vi "VisaReadExample2.vi"() -> ()   [LabVIEW 2016]
uses:
  <vilib>/Instr/_visa.llb/VISA Configure Serial Port (Instr).vi
panel:
  out "deleted portion":dbl[][](array[numeric])
  out "array w/ subset deleted":dbl[][](array[numeric])
  out "size(s)":i32
  out "PULSE":string="126526"
  in  "Upper Cut-Off":dbl=100.0
  in  "Lower Cut-Off":dbl=10.0
  in  "OK Button":bool
  out "Waveform Graph":dynamicdata(graph)
  in  "Array 2":dbl[](array[numeric])=array[6515 elements]
  in  "Array":dbl[](array[numeric])=array[6516 elements]
  out "substring 2":string="I"
  out "substring":string="126526"
  out "read buffer":string="I126526"
  in  "VISA resource name":refnum<visa-resource-name>="COM3"
  in  "stop":bool
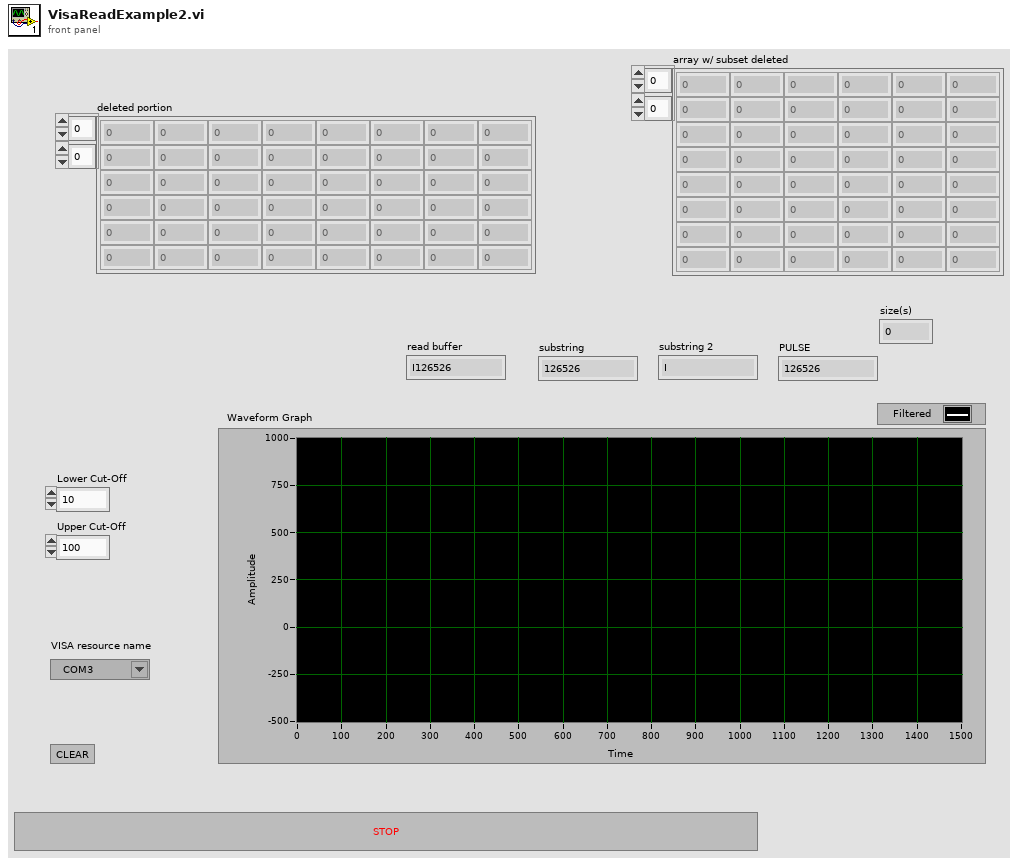
[diagram p1: front panel]
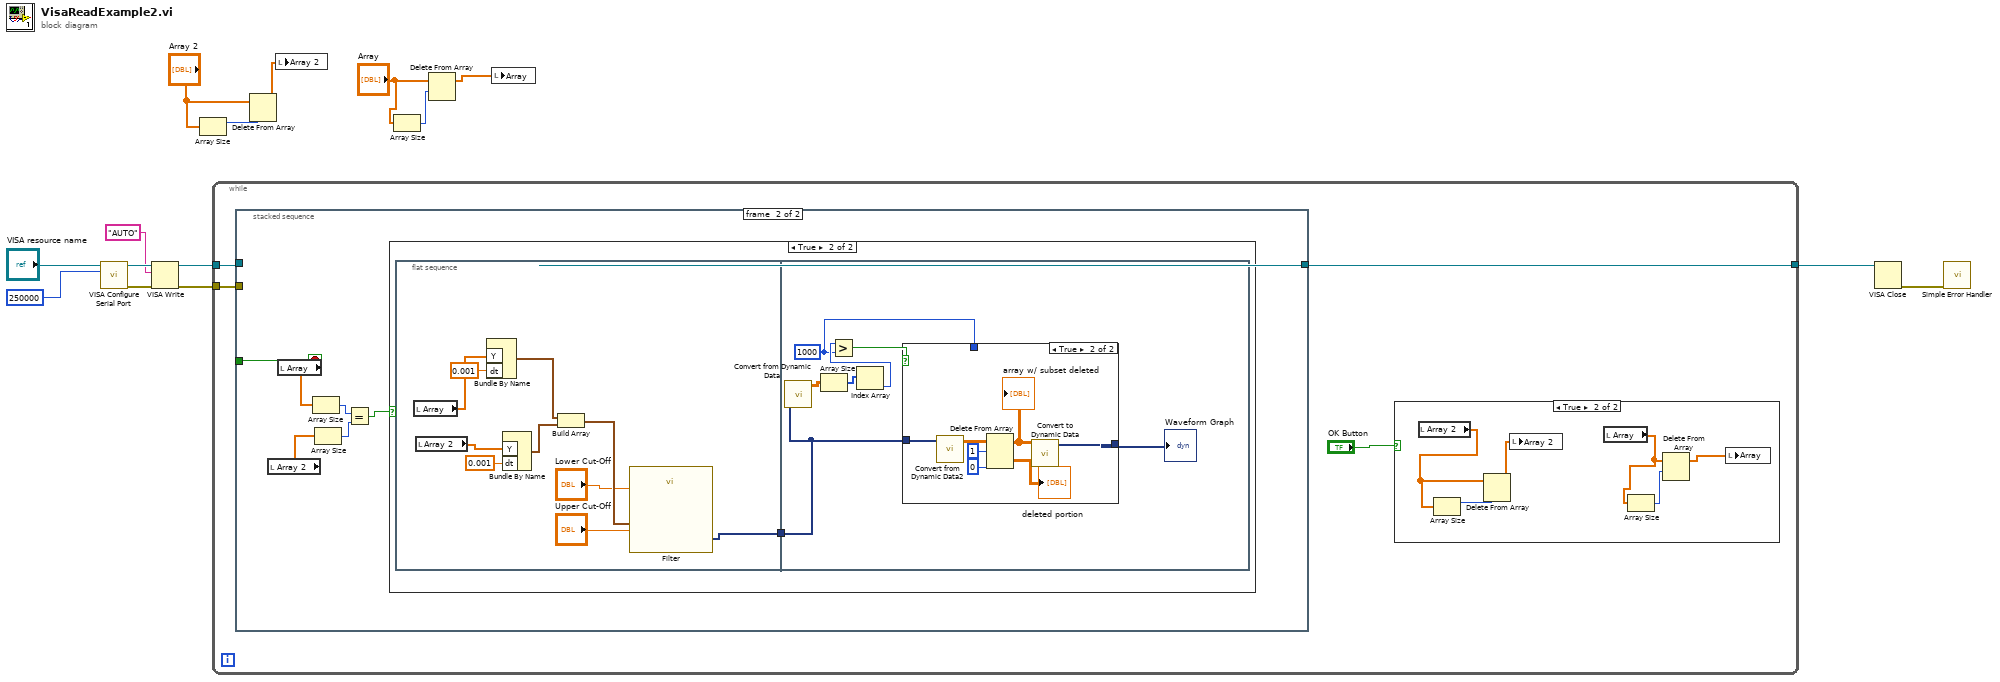
[diagram p0: block diagram]
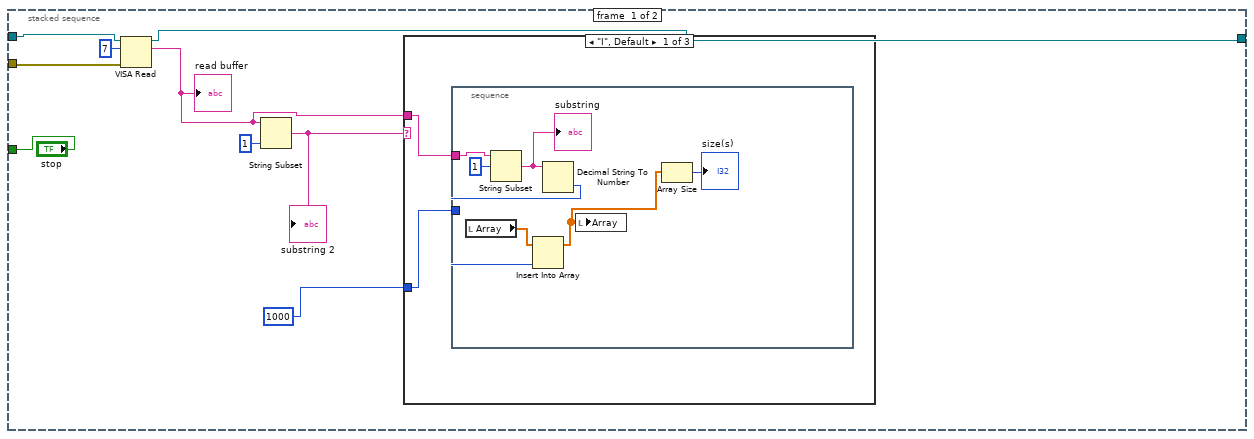
[diagram p3: hidden frame]
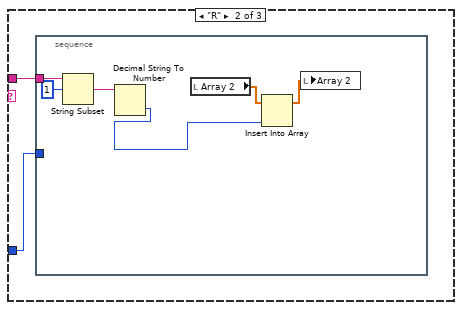
[diagram p4: hidden frame]
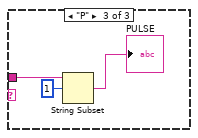
[diagram p5: hidden frame]
diagram:
  n1 = call-poly "VISA Configure Serial Port"("VISA resource name"="VISA resource name", "baud rate (9600)"=u32 250000) -> ("VISA resource name out"=w11:refnum<visa-resource-name>, "error out"=w9:errorcluster)  [unwired: 12 in]
  n2 = VISA Write(VISA resource name=w11, write buffer="AUTO", error in (no error)=w9) -> (VISA resource name out=w10:refnum<visa-resource-name>, error out=w8:errorcluster)  [unwired: 1 out]
  n3 = Array Size(array="Array 2") -> (size(s)=w3:i32)
  n4 = while {
    tunnel: [w19] -> w14
    tunnel: w10 -> [w18]
    tunnel: w8 -> [w17]
    stop <- w20 stop-if-true
    n5 = stacked-sequence {
      tunnel: ["stop" _] -> w20
      tunnel: [w34 _] -> w19
      tunnel: w18 -> [w32 _]
      tunnel: w17 -> [w29 _]
      frame #0 {
        n6 = VISA Read(VISA resource name=w32, byte count=u32 7, error in (no error)=w29) -> (VISA resource name out=w34:refnum<visa-resource-name>, read buffer=w28:string)  [unwired: 2 out]
        "read buffer" <- w28
        n7 = String Subset(string=w28, length (rest)=1 ("length (rest)")) -> (substring=w30:string)  [unwired: 1 in]
        "substring 2" <- w30
        n8 = case shown="\"I\", Default" w30 {
          tunnel: w28 -> [w37 w46 w53]
          tunnel: 1000 ("y") -> [w36 w45 _]
          frame "I", Default {
            n9 = stacked-sequence {
              tunnel: w37 -> [w43]
              tunnel: w36 -> [_]
              frame #0 {
                n10 = local read "Array"() -> (w41:dbl[])
                n11 = String Subset(string=w43, offset (0)=1) -> (substring=w42:string)  [unwired: 1 in]
                "substring" <- w42
                n12 = Decimal String To Number(string=w42) -> (number=w40:i32)  [unwired: 2 in, 1 out]
                n13 = Insert Into Array(array=w41, new element=w40) -> (w39:dbl[])  [unwired: 1 in]
                n14 = local write "Array"(w39) -> ()
                n15 = Array Size(array=w39) -> (size(s)=→"size(s)":i32)
              }
            }
          }
          frame "R" {
            n16 = stacked-sequence {
              tunnel: w46 -> [w52]
              tunnel: w45 -> [_]
              frame #0 {
                n17 = String Subset(string=w52, offset (0)=1) -> (substring=w50:string)  [unwired: 1 in]
                n18 = Decimal String To Number(string=w50) -> (number=w48:i32)  [unwired: 2 in, 1 out]
                n19 = local read "Array 2"() -> (w49:dbl[])
                n20 = Insert Into Array(array=w49, new element=w48) -> (w47:dbl[])  [unwired: 1 in]
                n21 = local write "Array 2"(w47) -> ()
              }
            }
          }
          frame "P" {
            n22 = String Subset(string=w53, offset (0)=1) -> (substring=→"PULSE":string)  [unwired: 1 in]
          }
        }
      }
      frame #1 {
        n23 = local read "Array 2"() -> (w60:dbl[])
        n24 = local read "Array"() -> (w59:dbl[])
        n25 = Array Size(array=w59) -> (size(s)=w58:i32)
        n26 = Array Size(array=w60) -> (size(s)=w57:i32)
        n27 = Equal?(x=w58, y=w57) -> (x = y?=w56:bool)
        n28 = case shown="True" w56 {
          frame False {
          }
          frame True {
            n29 = flat-sequence {
              tunnel: [w62] -> w61
              tunnel: w61 -> [w77]
              frame #0 {
                n30 = local read "Array"() -> (w71:dbl[])
                n31 = local read "Array 2"() -> (w70:dbl[])
                n32 = Bundle By Name("Y"=w71, "dt"=0.001) -> (w66:waveform(dbl))  [unwired: 1 in]
                n33 = Bundle By Name("Y"=w70, "dt"=0.001) -> (w67:waveform(dbl))  [unwired: 1 in]
                n34 = Build Array(w66, w67) -> (w65:waveform(dbl)[])
                n35 = call "Filter"("Lower Cut-Off"="Lower Cut-Off", "Upper Cut-Off"="Upper Cut-Off", "Signal"=w65) -> ("Filtered Signal"=w62:dynamicdata)  [unwired: 7 in, 1 out]
              }
              frame #1 {
                w73 = 1000 ("y")
                n36 = call "Convert from Dynamic Data"("Dynamic Data Type"=w77) -> ("Array"=w76:dbl[][])  [unwired: 3 in]
                n37 = Array Size(array=w76) -> (size(s)=w75:i32[])
                n38 = Index Array(array=w75) -> (element=w74:i32)  [unwired: 1 in]
                n39 = Greater?(x=w74, y=w73) -> (0:w78:bool)
                n40 = case shown="True" w78 {
                  tunnel: w77 -> [w79 w86]
                  tunnel: w73 -> [_ _]
                  tunnel: [w79 w82] -> w72
                  frame False {
                  }
                  frame True {
                    n41 = call "Convert from Dynamic Data2"("Dynamic Data Type"=w86) -> ("Array"=w85:dbl[][])  [unwired: 3 in]
                    n42 = Delete From Array(array=w85, length=1, index (row)=0) -> (deleted portion=→"deleted portion":dbl[][], array with subset deleted=w83:dbl[][])  [unwired: 1 in]
                    "array w/ subset deleted" <- w83
                    n43 = call "Convert to Dynamic Data"("2D Array"=w83) -> ("Dynamic Data Type"=w82:dynamicdata)  [unwired: 3 in]
                  }
                }
                "Waveform Graph" <- w72
              }
            }
          }
        }
      }
    }
    n44 = case shown="True" "OK Button" {
      frame False {
      }
      frame True {
        n45 = local read "Array 2"() -> (w22:dbl[])
        n46 = Array Size(array=w22) -> (size(s)=w25:i32)
        n47 = Delete From Array(array=w22, length=w25) -> (array with subset deleted=w24:dbl[])  [unwired: 1 in, 1 out]
        n48 = local write "Array 2"(w24) -> ()
        n49 = local read "Array"() -> (w21:dbl[])
        n50 = Array Size(array=w21) -> (size(s)=w26:i32)
        n51 = Delete From Array(array=w21, length=w26) -> (array with subset deleted=w23:dbl[])  [unwired: 1 in, 1 out]
        n52 = local write "Array"(w23) -> ()
      }
    }
  }
  n53 = Delete From Array(array="Array 2", length=w3) -> (array with subset deleted=w5:dbl[])  [unwired: 1 in, 1 out]
  n54 = local write "Array 2"(w5) -> ()
  n55 = Array Size(array="Array") -> (size(s)=w1:i32)
  n56 = Delete From Array(array="Array", length=w1) -> (array with subset deleted=w6:dbl[])  [unwired: 1 in, 1 out]
  n57 = local write "Array"(w6) -> ()
  n58 = VISA Close(VISA resource name=w14) -> (error out=w13:errorcluster)  [unwired: 1 in]
  n59 = call <vilib>:"Simple Error Handler.vi"("error in (no error)"=w13) -> ()  [unwired: 4 in, 5 out]
